vi "HTTP Headers to Map.vi"(11 "Headers":string) -> (3 "Map":map{string, string}(c390))   [LabVIEW 2020, in "GCentral-API.lvlib"]
uses:
  GCentral-API.lvlib
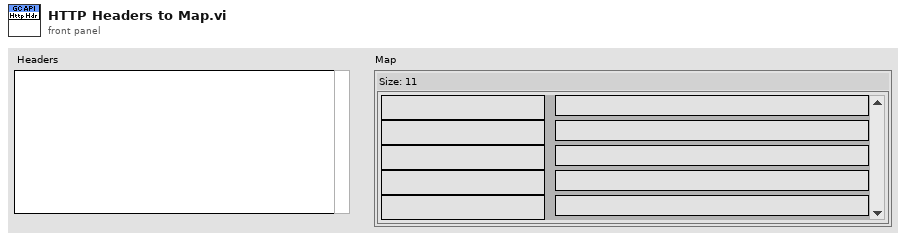
[diagram p1: front panel]
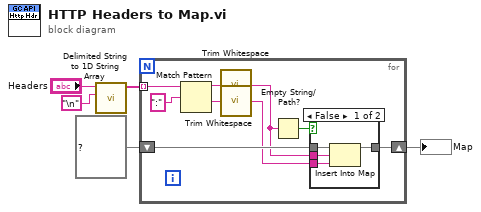
[diagram p0: block diagram]
diagram:
  n1 = call <vilib>:"Delimited String to 1D String Array.vi"("delimiter"="\n", "delimited string"="Headers") -> ("string array"=w3:string[])  [unwired: 9 in]
  n2 = for {
    tunnel: w3 -> [w9] mode=indexing
    shift-right: [w13] -> w1
    shift-left: map{string, string} {} ("Map") -> [w14]
    n3 = Match Pattern(string=w9, regular expression=":" ("delimiter")) -> (before substring=w7:string, after substring=w6:string)  [unwired: 1 in, 2 out]
    n4 = call <vilib>:"Trim Whitespace.vi"("string"=w7) -> ("trimmed string"=w10:string)  [unwired: 1 in]
    n5 = call <vilib>:"Trim Whitespace.vi"("string"=w6) -> ("trimmed string"=w12:string)  [unwired: 1 in]
    n6 = Empty String/Path?(string/path=w10) -> (empty?=w11:bool)
    n7 = case shown="False" w11 {
      tunnel: w14 -> [w18 w19]
      tunnel: w10 -> [w17 _]
      tunnel: [w16 w19] -> w13
      tunnel: w12 -> [w15 _]
      frame False {
        n8 = Insert Into Map(map in=w18, key=w17, value=w15) -> (map out=w16:map{string, string})  [unwired: 2 out]
      }
      frame True {
      }
    }
  }
  "Map" <- w1
